vi "Lift_State_Machine.vi"() -> ()   [LabVIEW 2016]
doc: "The state machine for the Lift System.\nDrives the lift forward, then upward, then back, then down to its origin."
uses:
  <vilib>/myRIO/Instrument Drivers/Onboard IO/DIO/typedefs/DIO Reference.ctl
  <vilib>/myRIO/Common/Instrument Driver Framework/Utilities/typedefs/myRIO Generic Hardware Reference.ctl
  <vilib>/myRIO/Common/Instrument Driver Framework/Utilities/typedefs/Hardware Version Enum.ctl
  <vilib>/myRIO/Common/Instrument Driver Framework/Utilities/typedefs/myRIO v1.0 Reference.ctl
  <vilib>/myRIO/Common/Instrument Driver Framework/Utilities/typedefs/Generic FPGA Reference.ctl
  <vilib>/myRIO/Common/Instrument Driver Framework/myRIO v1.0/DIO/typedefs/DIO Channels List.ctl
  <vilib>/myRIO/Common/Instrument Driver Framework/myRIO v1.0/DIO/typedefs/DIO Channels Enum.ctl
  <vilib>/userdefined/High Color/nirio_resource_hc.ctl
  <vilib>/myRIO/Common/Instrument Driver Framework/Utilities/vis/Is FPGA Ref Available.vi
  <vilib>/myRIO/Common/Instrument Driver Framework/roboRIO v1.0/DIO/vis/roboRIO v1.0 Open DIO.vi
  <vilib>/myRIO/Instrument Drivers/Onboard IO/DIO/vis/Write.vi
  <vilib>/myRIO/Instrument Drivers/Onboard IO/DIO/vis/Read.vi
  <vilib>/myRIO/Common/Instrument Driver Framework/Utilities/vis/Validate Channels.vi
  <vilib>/myRIO/Common/Instrument Driver Framework/roboRIO v1.0/DIO/vis/roboRIO v1.0 Reserve DIO.vi
  <vilib>/myRIO/Common/Instrument Driver Framework/roboRIO v1.0/DIO/vis/roboRIO v1.0 Build MUX Configuration DIO.vi
  <vilib>/myRIO/Common/Instrument Driver Framework/roboRIO v1.0/Resource Manager/vis/roboRIO v1.0 Reserve Channel List.vi
  <vilib>/myRIO/Common/Instrument Driver Framework/roboRIO v1.0/Resource Manager/vis/roboRIO v1.0 Create Configuration List.vi
  <vilib>/myRIO/Common/Instrument Driver Framework/roboRIO v1.0/Resource Manager/vis/roboRIO v1.0 Reserve Channel.vi
  <vilib>/myRIO/Common/Instrument Driver Framework/roboRIO v1.0/Resource Manager/vis/roboRIO v1.0 Unreserve Channel.vi
  <vilib>/myRIO/Common/Instrument Driver Framework/roboRIO v1.0/Resource Manager/vis/roboRIO v1.0 Build Mutex Name.vi
  GlobalVI.vi
  <vilib>/Utility/VariantDataType/GetNumericInfo.vi
  <vilib>/Utility/error.llb/Error Cluster From Error Code.vi
  <vilib>/myRIO/Common/Instrument Driver Framework/roboRIO v1.0/roboRIO v1.0 Open.vi
  <vilib>/myRIO/Common/Instrument Driver Framework/Utilities/vis/IO Manager.vi
  <vilib>/myRIO/Common/Instrument Driver Framework/Utilities/vis/Configuration Manager.vi
  <vilib>/myRIO/Common/Instrument Driver Framework/roboRIO v1.0/Resource Manager/vis/roboRIO v1.0 Configure IO.vi
  <vilib>/myRIO/Common/Instrument Driver Framework/myRIO v1.0/myRIO v1.0 Close.vi
  <vilib>/myRIO/Common/Instrument Driver Framework/roboRIO v1.0/DIO/vis/roboRIO v1.0 Read DIO.vi
  <vilib>/myRIO/Common/Instrument Driver Framework/roboRIO v1.0/DIO/vis/roboRIO v1.0 Write DIO.vi
  <vilib>/myRIO/Express VI/Onboard IO/DI/DI Express VI.xnode
  <vilib>/myRIO/Instrument Drivers/Onboard IO/DIO/vis/myRIO DIO Open.xnode
  <vilib>/myRIO/Express VI/Onboard IO/DO/DO Express VI.xnode
  <vilib>/myRIO/Express VI/Onboard Devices/LED/LED Express VI.xnode
  <vilib>/myRIO/Instrument Drivers/Onboard IO/DIO/DIO.lvlib
panel:
  out "DIO/DIO4 (Pin 4)":bool
  out "TrashCanOn":bool
  out "Trash can detection)":bool
  out "B/DIO7 (Pin 25) 4":bool
  out "B/DIO9 (Pin 29) 4":bool
  out "B/DIO8 (Pin 27) 4":bool
  out "B/DIO7 (Pin 25)":bool
  out "B/DIO8 (Pin 27)":bool
  out "B/DIO9 (Pin 29) 2":bool
  in  "runLiftStatemachine":bool
  out "timeoutError":bool
  out "timeoutCounter":u32
  out "timerCount":u32
  out "liftState":i32
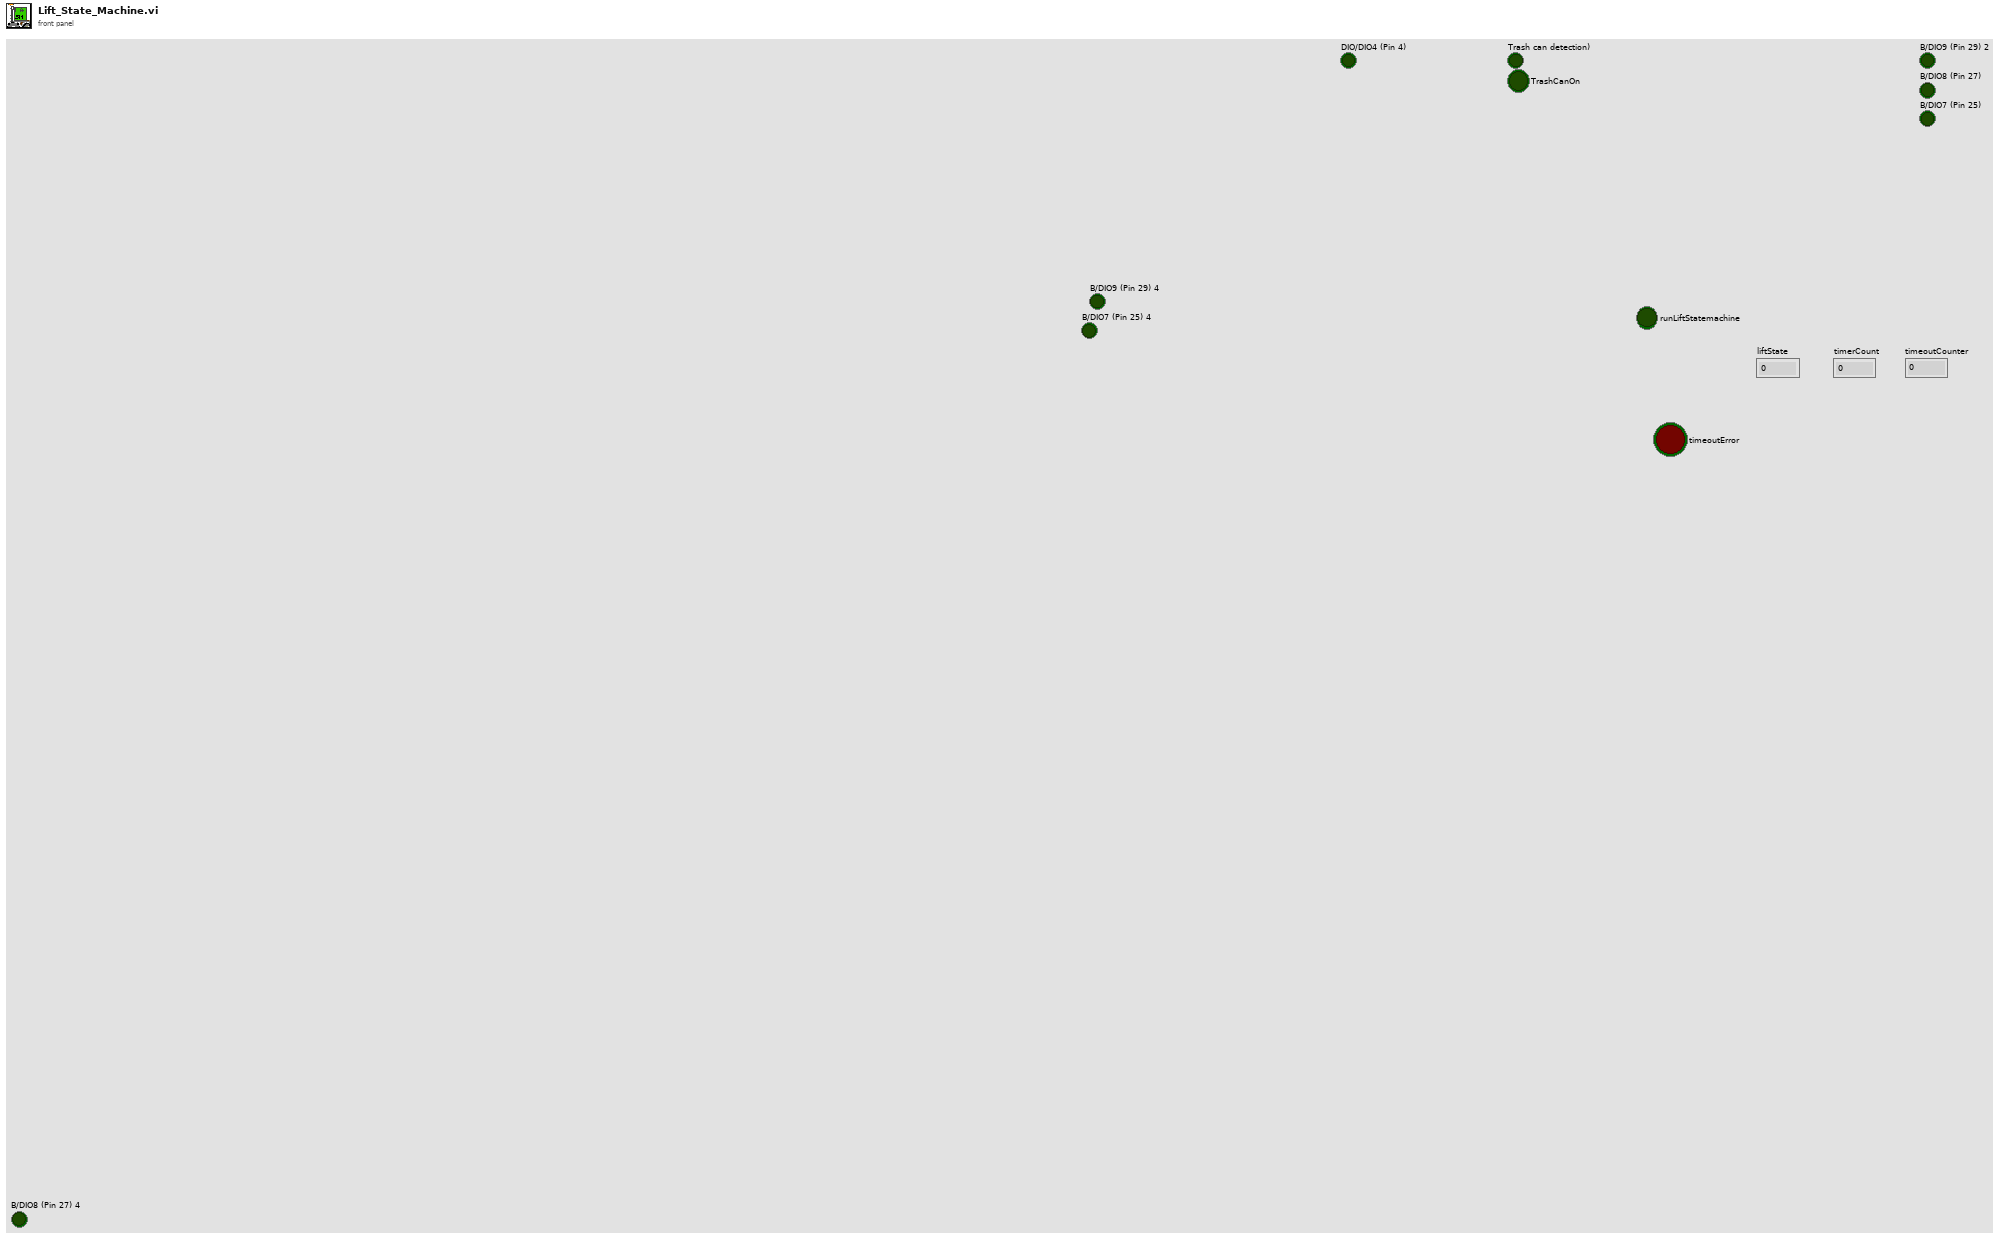
[diagram p1: front panel]
types:
  T1 = typedef "DIO.lvlib/DIO Reference.ctl" = cluster{"myRIO Reference":T2, "DIO Channels List":T6}
  T2 = typedef "myRIO Generic Hardware Reference.ctl" = cluster{"myRIO Model":T3, "myRIO Hardware Reference":T4}
  T3 = typedef "Hardware Version Enum.ctl" = enum16{"Unknown", "myRIO-1900", "myRIO-1950", "roboRIO", "NI ELVIS RIO CM"}
  T4 = typedef "myRIO v1.0 Reference.ctl" = cluster{"Generic FPGA Reference":T5, "Allow multiple opens":bool}
  T5 = typedef "Generic FPGA Reference.ctl" = refnum<k20>
  T6 = typedef "DIO Channels List.ctl" = T7[]
  T7 = typedef "DIO Channels Enum.ctl" = enum16{"Not Connected", "C/DIO0", "C/DIO1", "C/DIO2", "C/DIO3", "C/DIO4", "C/DIO5", "C/DIO6", "C/DIO7", "A/DIO0", "A/DIO1", "A/DIO2", "A/DIO3", "A/DIO4", "A/DIO5", "A/DIO6", "A/DIO7", "A/DIO8", "A/DIO9", "A/DIO10", "A/DIO11", "A/DIO12", "A/DIO13", "A/DIO14", "A/DIO15", "B/DIO0", "B/DIO1", "B/DIO2", "B/DIO3", "B/DIO4", "B/DIO5", "B/DIO6", "B/DIO7", "B/DIO8", "B/DIO9", "B/DIO10", "B/DIO11", "B/DIO12", "B/DIO13", "B/DIO14", "B/DIO15", "LED0", "LED1", "LED2", "LED3", "Button0", "DIO/DIO0", "DIO/DIO1", "DIO/DIO2", "DIO/DIO3", "DIO/DIO4", "DIO/DIO5", "DIO/DIO6", "DIO/DIO7", "DIO/DIO8", "DIO/DIO9", "SPI/CS0", "SPI/CS1", "SPI/CS2", "SPI/CS3", "LED RADIO (Green)", "LED RADIO (Red)", "LED COMM (Green)", "LED COMM (Red)", "LED MODE (Green)", "LED MODE (Red)"}
  T8 = typedef "nirio_resource_hc.ctl" = tag
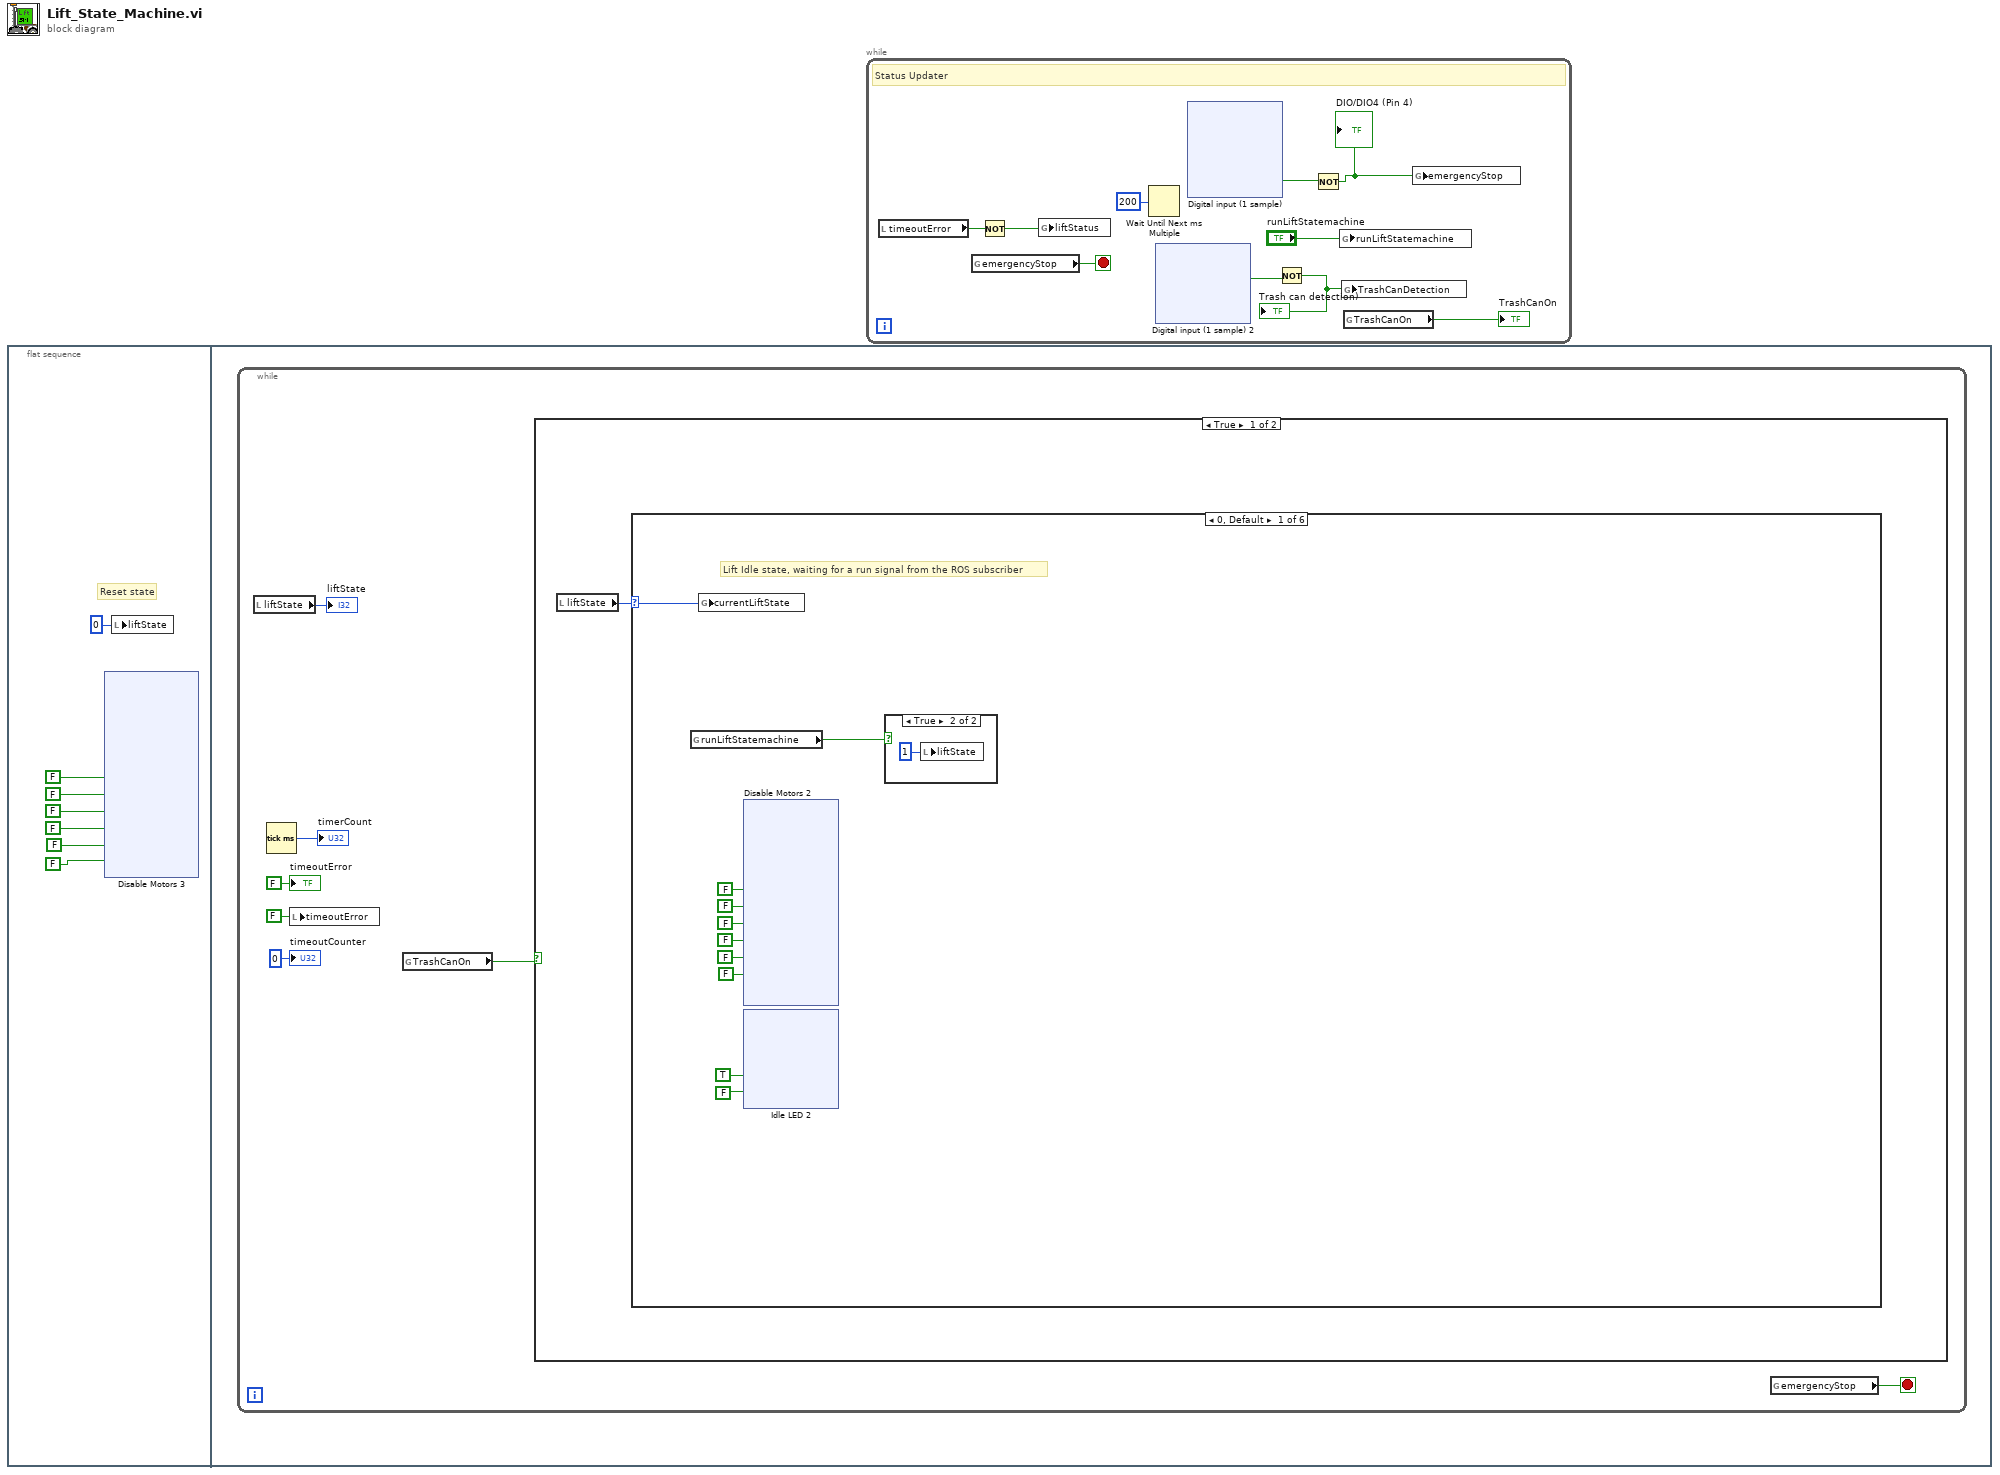
[diagram p0: block diagram]
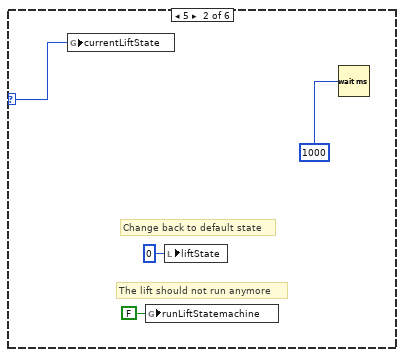
[diagram p3: hidden frame]
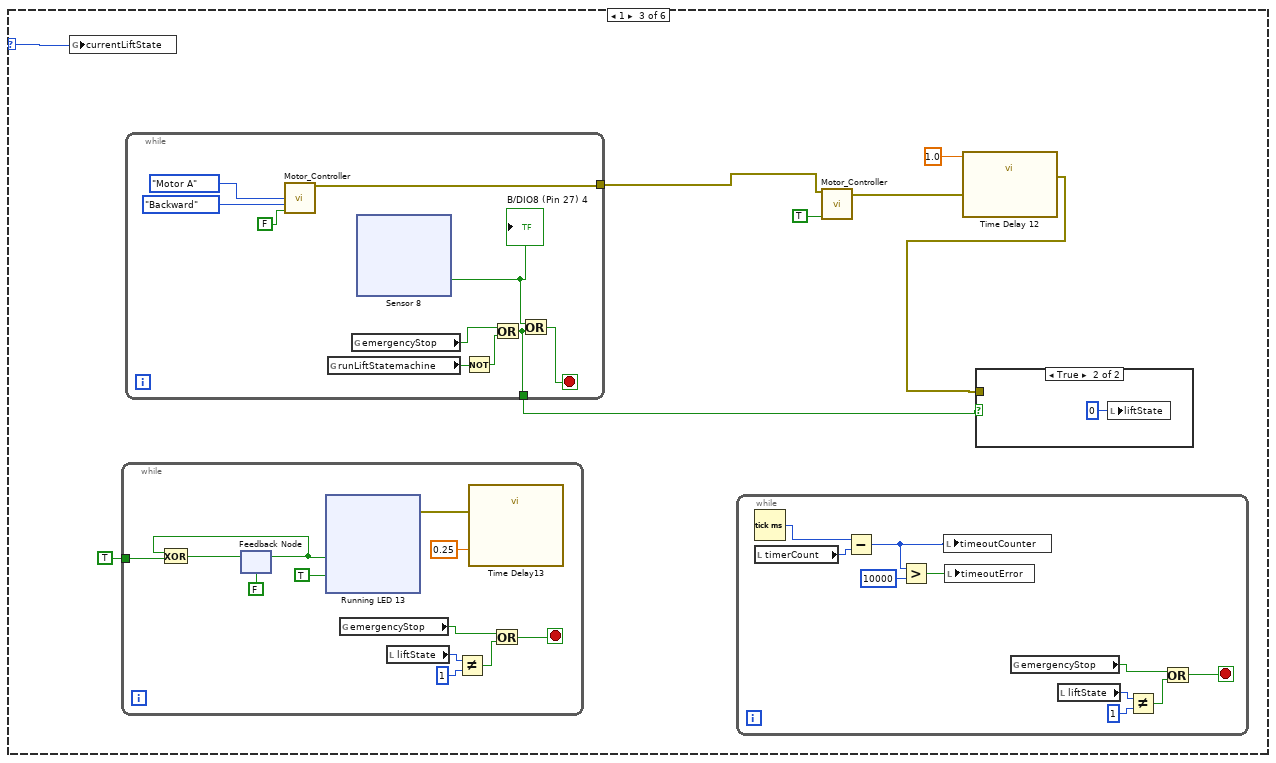
[diagram p4: hidden frame]
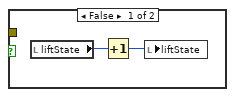
[diagram p5: hidden frame]
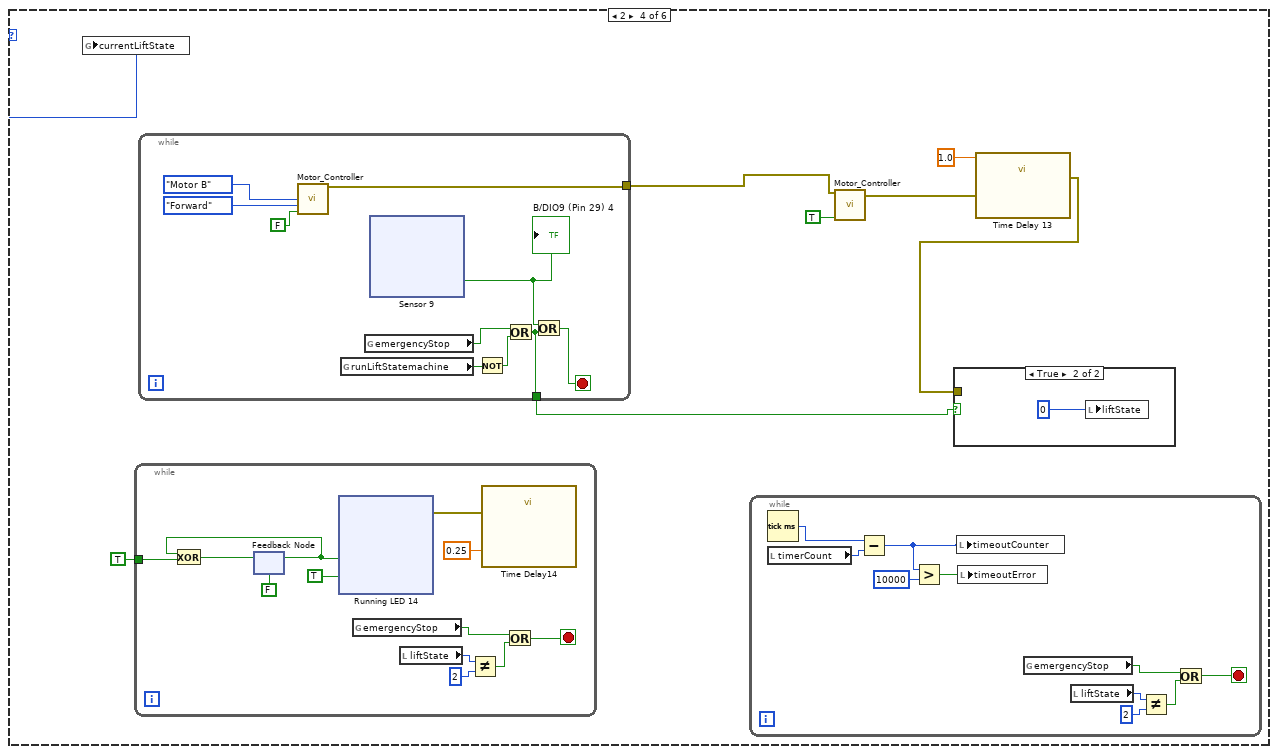
[diagram p6: hidden frame]
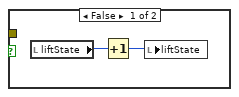
[diagram p7: hidden frame]
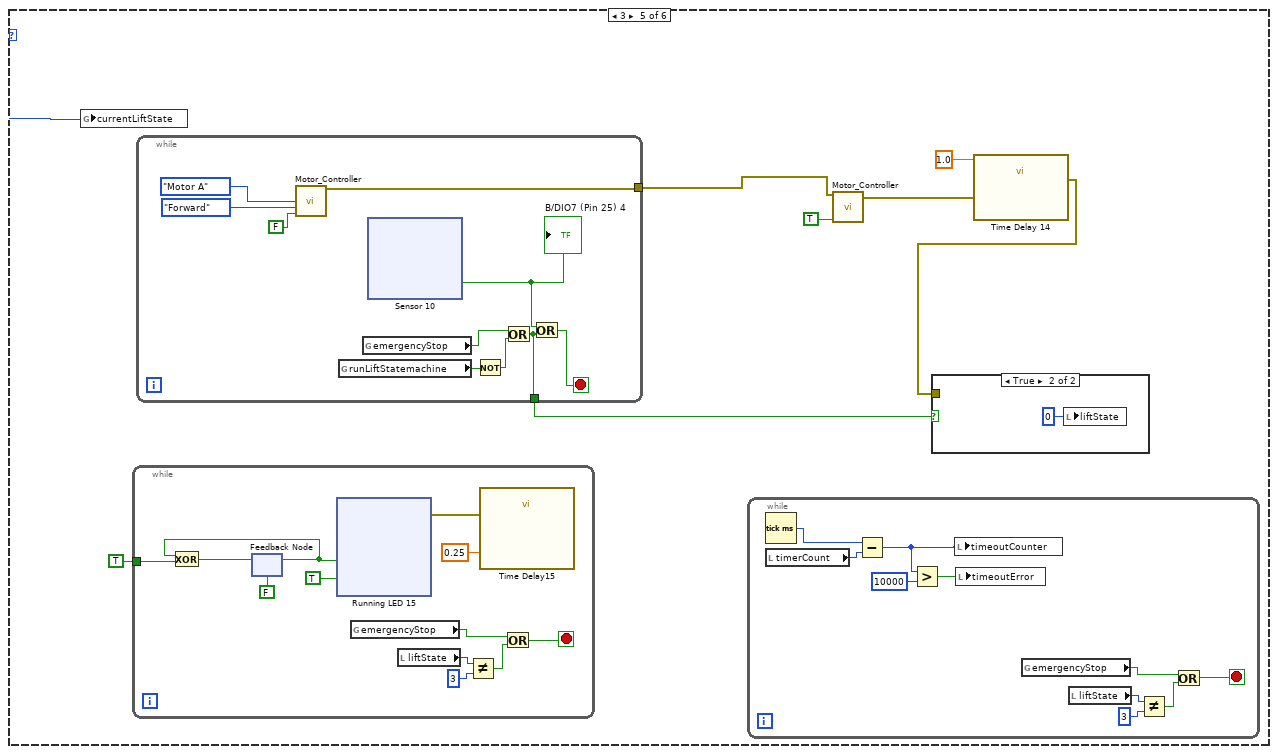
[diagram p8: hidden frame]
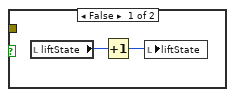
[diagram p9: hidden frame]
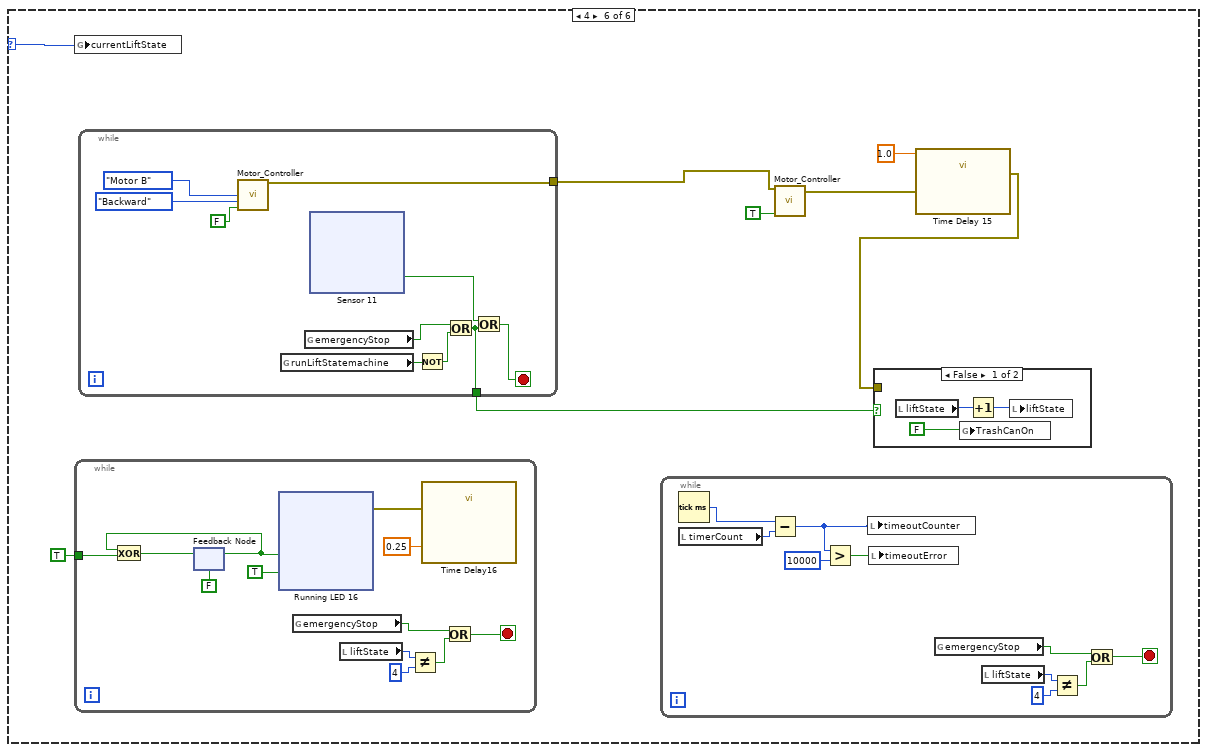
[diagram p10: hidden frame]
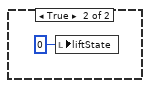
[diagram p11: hidden frame]
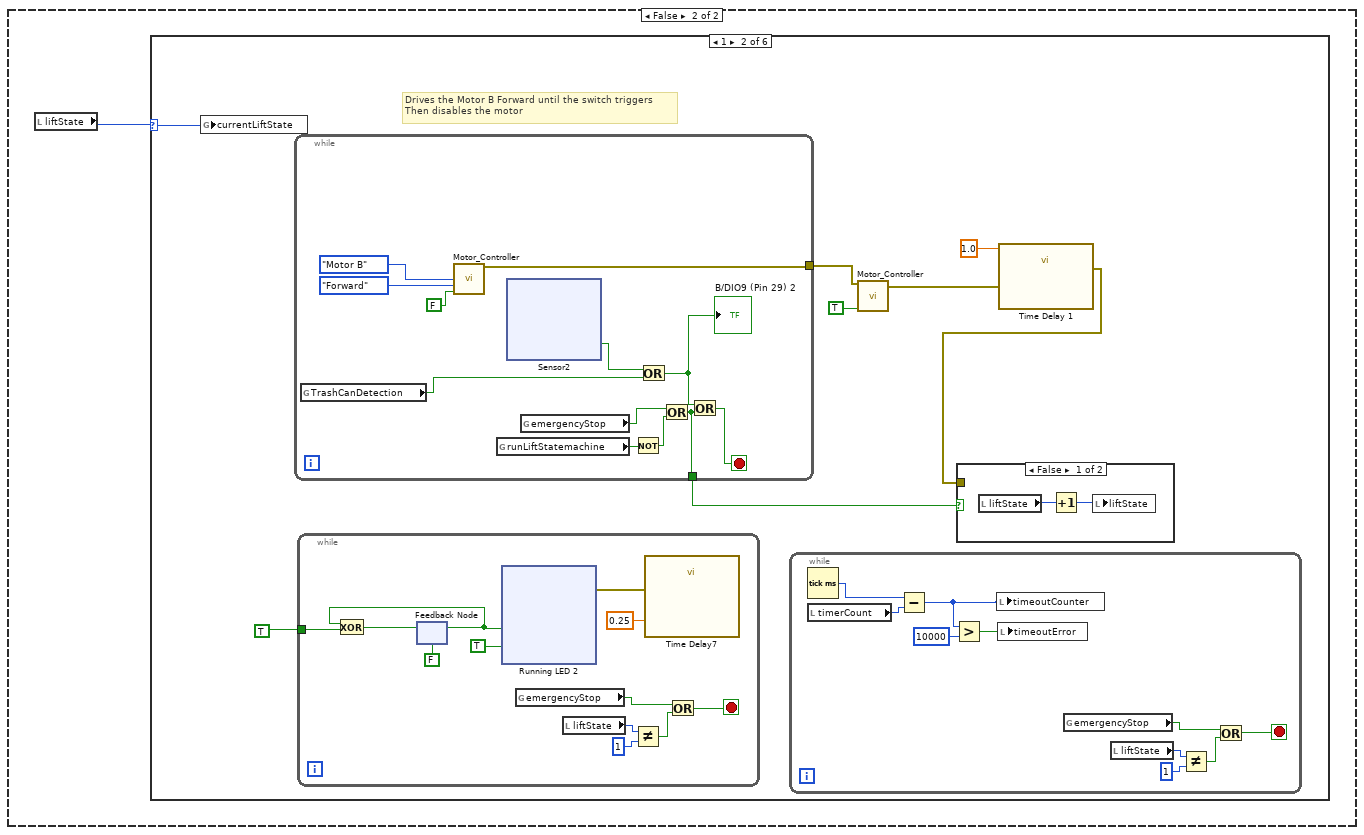
[diagram p12: hidden frame]
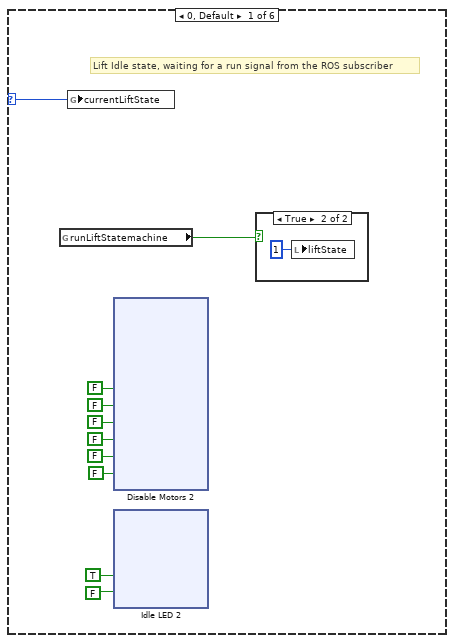
[diagram p13: hidden frame]
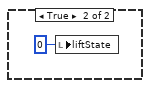
[diagram p15: hidden frame]
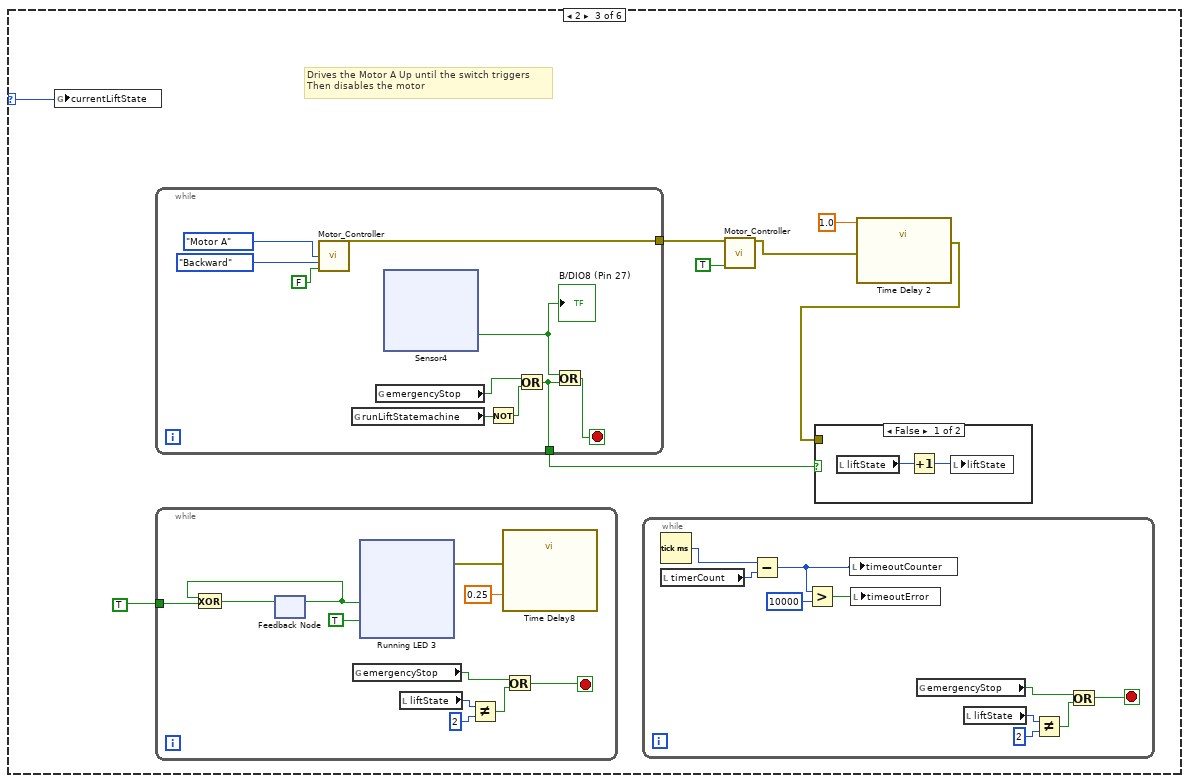
[diagram p16: hidden frame]
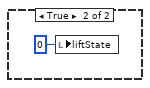
[diagram p17: hidden frame]
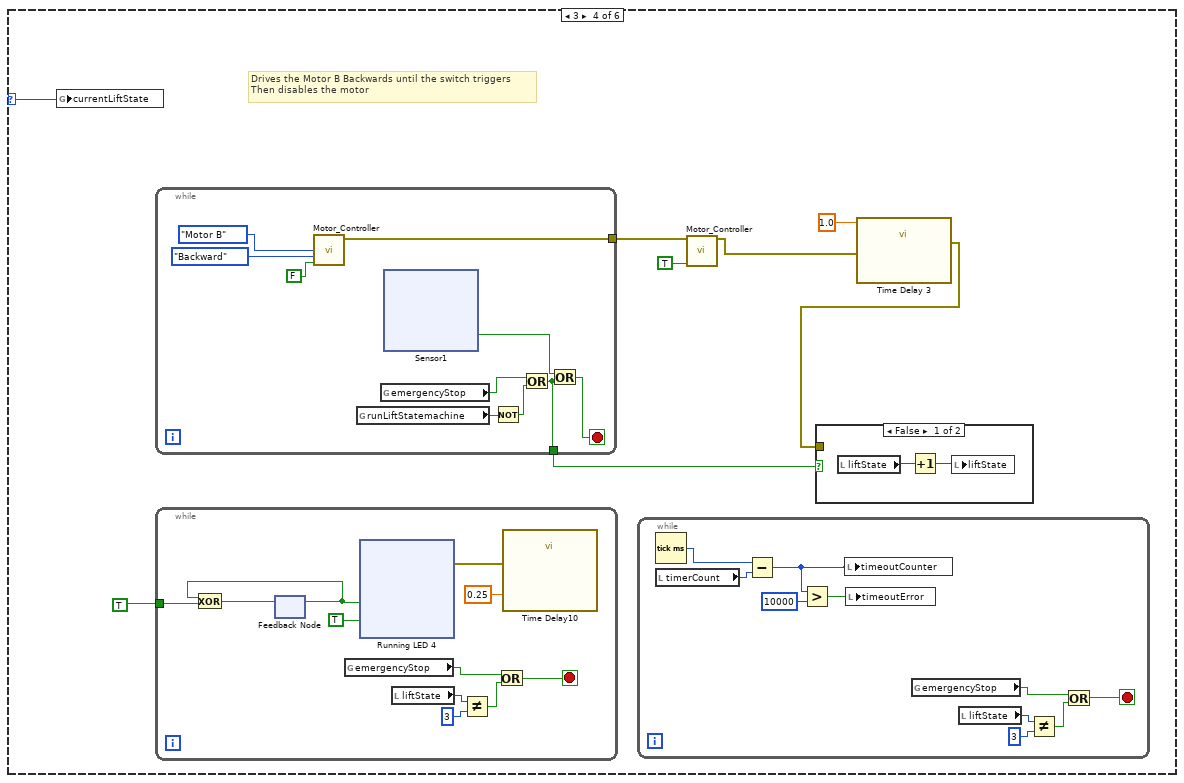
[diagram p18: hidden frame]
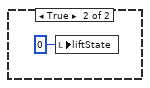
[diagram p19: hidden frame]
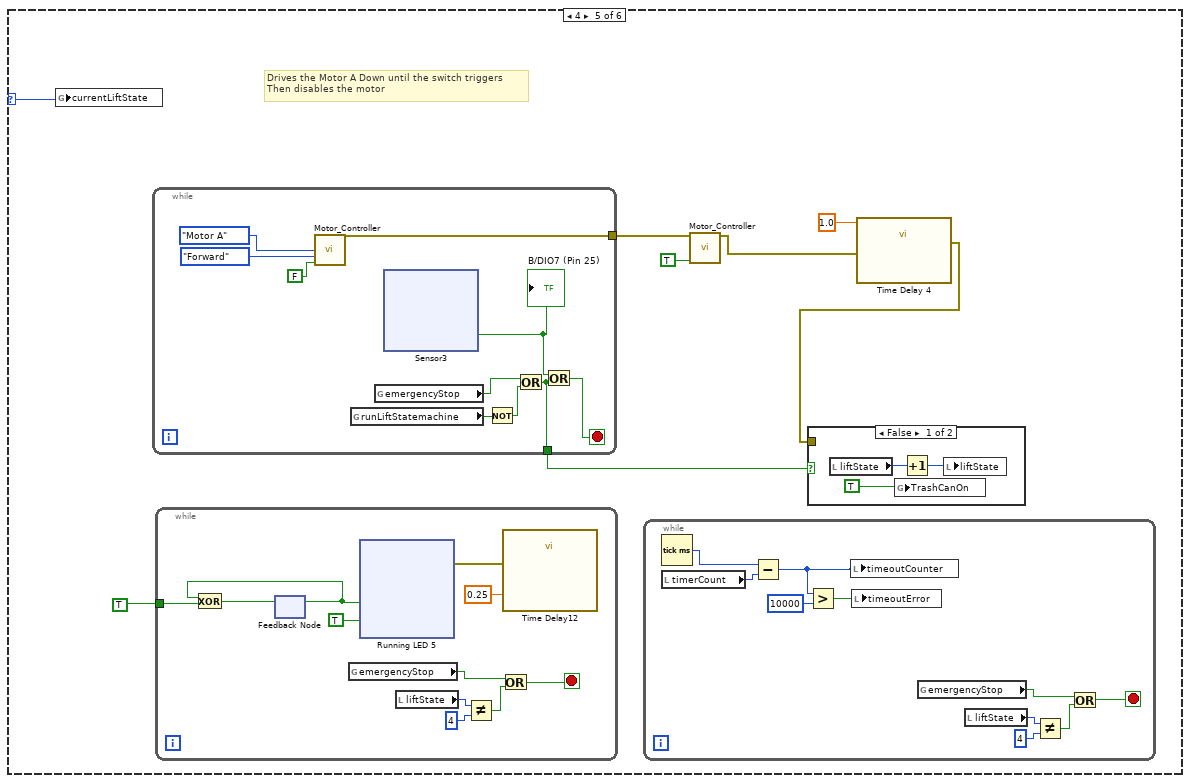
[diagram p20: hidden frame]
diagram:
  n1 = flat-sequence {
    frame #0 {
      # "Reset state"
      n2 = xnode "Disable Motors 3"("IN1 (B/DIO0 (Pin 11))"=FALSE ("IN2 (B/DIO1 (Pin 13))"), "IN2 (B/DIO1 (Pin 13))"=FALSE ("IN3 (B/DIO2 (Pin 15))"), "IN3 (B/DIO2 (Pin 15))"=FALSE ("IN4 (B/DIO3 (Pin 17))"), "IN4 (B/DIO3 (Pin 17))"=FALSE ("ENABLE A (B/DIO13 (Pin 26))"), "ENABLE A (B/DIO13 (Pin 26))"=FALSE ("ENABLE B (B/DIO8 (Pin 27))"), "ENABLE B (B/DIO8 (Pin 27))"=FALSE) -> ()  [unwired: 1 in, 1 out]
      n3 = local write "liftState"(0 ("liftState")) -> ()
    }
    frame #1 {
      n4 = while {
        stop <- w54 stop-if-true
        n5 = local read "liftState"() -> (→"liftState":i32)
        n6 = Tick Count (ms)() -> (millisecond timer value=→"timerCount":u32)
        n7 = local write "timeoutError"(FALSE ("timeoutError")) -> ()
        n8 = global read "GlobalVI.vi" "TrashCanOn"() -> (w48:bool)
        n9 = case shown="True" w48 {
          frame True {
            n10 = local read "liftState"() -> (w55:i32)
            n11 = case shown="0, Default" w55 {
              selector: w55 -> [w56 w145 w154 w263 w375 w489]
              frame 0, Default {
                # "Lift Idle state, waiting for a run signal from the ROS subscriber"
                n12 = global read "GlobalVI.vi" "runLiftStatemachine"() -> (w57:bool)
                n13 = global write "GlobalVI.vi" "currentLiftState"(w56) -> ()
                n14 = xnode "Disable Motors 2"("IN1 (B/DIO0 (Pin 11))"=FALSE, "IN2 (B/DIO1 (Pin 13))"=FALSE, "IN3 (B/DIO2 (Pin 15))"=FALSE, "IN4 (B/DIO3 (Pin 17))"=FALSE, "ENABLE A (B/DIO13 (Pin 26))"=FALSE, "ENABLE B (B/DIO8 (Pin 27))"=FALSE) -> ()  [unwired: 1 in, 1 out]
                n15 = xnode "Idle LED 2"("CommG"=TRUE, "CommR"=FALSE ("CommG")) -> ()  [unwired: 1 in, 1 out]
                n16 = case shown="True" w57 {
                  frame False {
                  }
                  frame True {
                    n17 = local write "liftState"(1 ("liftState")) -> ()
                  }
                }
              }
              frame 5 {
                # "The lift should not run anymore"
                # "Change back to default state"
                n18 = global write "GlobalVI.vi" "currentLiftState"(w145) -> ()
                n19 = global write "GlobalVI.vi" "runLiftStatemachine"(FALSE ("runLiftStatemachine")) -> ()
                n20 = local write "liftState"(0 ("liftState")) -> ()
                n21 = Wait (ms)(milliseconds to wait=u32 1000) -> ()  [unwired: 1 out]
              }
              frame 1 {
                n22 = global write "GlobalVI.vi" "currentLiftState"(w154) -> ()
                n23 = while {
                  tunnel: TRUE ("COMM (Red)") -> [w179]
                  stop <- w169 stop-if-true
                  n24 = feedback #1(FALSE) -> (w177:bool)
                  n25 = Exclusive Or(1:w179, 2:w177) -> (0:w178:bool)
                  n26 = feedback-in #1(w178) -> ()
                  n27 = xnode "Running LED 13"("CommG"=w177, "CommR"=TRUE) -> ("error out"=w174:errorcluster)  [unwired: 1 in]
                  n28 = global read "GlobalVI.vi" "emergencyStop"() -> (w170:bool)
                  n29 = local read "liftState"() -> (w172:i32)
                  n30 = Not Equal?(x=w172, y=1 ("liftState")) -> (x != y?=w171:bool)
                  n31 = call "Time Delay13"("error in (no error)"=w174, "Delay Time (s)"=0.25) -> ()  [unwired: 9 in, 1 out]
                  n32 = Or(x=w170, y=w171) -> (x .or. y?=w169:bool)
                }
                n33 = while {
                  tunnel: [w220] -> w149
                  tunnel: [w221] -> w147
                  stop <- w225 stop-if-true
                  n34 = call "Motor_Controller.vi"("motorSelect"=enum16{"Motor A", "Motor B"}."Motor A", "direction"=enum16{"Forward", "Backward"}."Backward", "stopMotors"=FALSE) -> ("error out"=w220:errorcluster)  [unwired: 12 in]
                  n35 = global read "GlobalVI.vi" "runLiftStatemachine"() -> (w224:bool)
                  n36 = global read "GlobalVI.vi" "emergencyStop"() -> (w222:bool)
                  n37 = xnode "Sensor 8"() -> ("B/DIO8 (Pin 27)"=w216:bool)  [unwired: 1 in, 1 out]
                  "B/DIO8 (Pin 27) 4" <- w216
                  n38 = Not(x=w224) -> (.not. x?=w223:bool)
                  n39 = Or(x=w222, y=w223) -> (x .or. y?=w221:bool)
                  n40 = Or(x=w216, y=w221) -> (x .or. y?=w225:bool)
                }
                n41 = while {
                  stop <- w161 stop-if-true
                  n42 = Tick Count (ms)() -> (millisecond timer value=w167:u32)
                  n43 = local read "timerCount"() -> (w166:u32)
                  n44 = Subtract(x=w167, y=w166) -> (x-y=w158:u32)
                  n45 = Greater?(x=w158, y=u32 10000) -> (0:w159:bool)
                  n46 = local write "timeoutCounter"(w158) -> ()
                  n47 = local write "timeoutError"(w159) -> ()
                  n48 = global read "GlobalVI.vi" "emergencyStop"() -> (w165:bool)
                  n49 = local read "liftState"() -> (w163:i32)
                  n50 = Not Equal?(x=w163, y=1 ("liftState")) -> (x != y?=w164:bool)
                  n51 = Or(x=w165, y=w164) -> (x .or. y?=w161:bool)
                }
                n52 = call "Motor_Controller.vi"("error in (no error)"=w149, "stopMotors"=TRUE) -> ("error out"=w150:errorcluster)  [unwired: 13 in]
                n53 = call "Time Delay 12"("error in (no error)"=w150, "Delay Time (s)"=1.0) -> ("error out"=w148:errorcluster)  [unwired: 9 in]
                n54 = case shown="True" w147 {
                  tunnel: w148 -> [_ _]
                  frame False {
                    n55 = local read "liftState"() -> (w156:i32)
                    n56 = Increment(x=w156) -> (x+1=w155:i32)
                    n57 = local write "liftState"(w155) -> ()
                  }
                  frame True {
                    n58 = local write "liftState"(0 ("liftState")) -> ()
                  }
                }
              }
              frame 2 {
                n59 = global write "GlobalVI.vi" "currentLiftState"(w263) -> ()
                n60 = while {
                  tunnel: TRUE ("COMM (Red)") -> [w293]
                  stop <- w283 stop-if-true
                  n61 = feedback #2(FALSE) -> (w291:bool)
                  n62 = Exclusive Or(1:w293, 2:w291) -> (0:w292:bool)
                  n63 = feedback-in #2(w292) -> ()
                  n64 = xnode "Running LED 14"("CommG"=w291, "CommR"=TRUE) -> ("error out"=w288:errorcluster)  [unwired: 1 in]
                  n65 = global read "GlobalVI.vi" "emergencyStop"() -> (w284:bool)
                  n66 = local read "liftState"() -> (w286:i32)
                  n67 = Not Equal?(x=w286, y=2 ("liftState")) -> (x != y?=w285:bool)
                  n68 = call "Time Delay14"("error in (no error)"=w288, "Delay Time (s)"=0.25) -> ()  [unwired: 9 in, 1 out]
                  n69 = Or(x=w284, y=w285) -> (x .or. y?=w283:bool)
                }
                n70 = while {
                  tunnel: [w334] -> w264
                  tunnel: [w335] -> w261
                  stop <- w339 stop-if-true
                  n71 = call "Motor_Controller.vi"("motorSelect"=enum16{"Motor A", "Motor B"}."Motor B", "direction"=enum16{"Forward", "Backward"}."Forward", "stopMotors"=FALSE) -> ("error out"=w334:errorcluster)  [unwired: 12 in]
                  n72 = global read "GlobalVI.vi" "runLiftStatemachine"() -> (w338:bool)
                  n73 = global read "GlobalVI.vi" "emergencyStop"() -> (w336:bool)
                  n74 = xnode "Sensor 9"() -> ("B/DIO9 (Pin 29)"=w330:bool)  [unwired: 1 in, 1 out]
                  "B/DIO9 (Pin 29) 4" <- w330
                  n75 = Not(x=w338) -> (.not. x?=w337:bool)
                  n76 = Or(x=w336, y=w337) -> (x .or. y?=w335:bool)
                  n77 = Or(x=w330, y=w335) -> (x .or. y?=w339:bool)
                }
                n78 = while {
                  stop <- w275 stop-if-true
                  n79 = Tick Count (ms)() -> (millisecond timer value=w281:u32)
                  n80 = local read "timerCount"() -> (w280:u32)
                  n81 = Subtract(x=w281, y=w280) -> (x-y=w272:u32)
                  n82 = Greater?(x=w272, y=u32 10000) -> (0:w273:bool)
                  n83 = local write "timeoutCounter"(w272) -> ()
                  n84 = local write "timeoutError"(w273) -> ()
                  n85 = global read "GlobalVI.vi" "emergencyStop"() -> (w279:bool)
                  n86 = local read "liftState"() -> (w277:i32)
                  n87 = Not Equal?(x=w277, y=2 ("liftState")) -> (x != y?=w278:bool)
                  n88 = Or(x=w279, y=w278) -> (x .or. y?=w275:bool)
                }
                n89 = call "Motor_Controller.vi"("error in (no error)"=w264, "stopMotors"=TRUE) -> ("error out"=w265:errorcluster)  [unwired: 13 in]
                n90 = call "Time Delay 13"("error in (no error)"=w265, "Delay Time (s)"=1.0) -> ("error out"=w262:errorcluster)  [unwired: 9 in]
                n91 = case shown="True" w261 {
                  tunnel: w262 -> [_ _]
                  frame False {
                    n92 = local read "liftState"() -> (w270:i32)
                    n93 = Increment(x=w270) -> (x+1=w269:i32)
                    n94 = local write "liftState"(w269) -> ()
                  }
                  frame True {
                    n95 = local write "liftState"(0 ("liftState")) -> ()
                  }
                }
              }
              frame 3 {
                n96 = global write "GlobalVI.vi" "currentLiftState"(w375) -> ()
                n97 = while {
                  tunnel: TRUE ("COMM (Red)") -> [w407]
                  stop <- w397 stop-if-true
                  n98 = feedback #3(FALSE) -> (w405:bool)
                  n99 = Exclusive Or(1:w407, 2:w405) -> (0:w406:bool)
                  n100 = feedback-in #3(w406) -> ()
                  n101 = xnode "Running LED 15"("CommG"=w405, "CommR"=TRUE) -> ("error out"=w402:errorcluster)  [unwired: 1 in]
                  n102 = global read "GlobalVI.vi" "emergencyStop"() -> (w398:bool)
                  n103 = local read "liftState"() -> (w400:i32)
                  n104 = Not Equal?(x=w400, y=3 ("liftState")) -> (x != y?=w399:bool)
                  n105 = call "Time Delay15"("error in (no error)"=w402, "Delay Time (s)"=0.25) -> ()  [unwired: 9 in, 1 out]
                  n106 = Or(x=w398, y=w399) -> (x .or. y?=w397:bool)
                }
                n107 = while {
                  tunnel: [w448] -> w377
                  tunnel: [w449] -> w376
                  stop <- w453 stop-if-true
                  n108 = call "Motor_Controller.vi"("motorSelect"=enum16{"Motor A", "Motor B"}."Motor A", "direction"=enum16{"Forward", "Backward"}."Forward", "stopMotors"=FALSE) -> ("error out"=w448:errorcluster)  [unwired: 12 in]
                  n109 = global read "GlobalVI.vi" "runLiftStatemachine"() -> (w452:bool)
                  n110 = global read "GlobalVI.vi" "emergencyStop"() -> (w450:bool)
                  n111 = xnode "Sensor 10"() -> ("B/DIO7 (Pin 25)"=w444:bool)  [unwired: 1 in, 1 out]
                  "B/DIO7 (Pin 25) 4" <- w444
                  n112 = Not(x=w452) -> (.not. x?=w451:bool)
                  n113 = Or(x=w450, y=w451) -> (x .or. y?=w449:bool)
                  n114 = Or(x=w444, y=w449) -> (x .or. y?=w453:bool)
                }
                n115 = while {
                  stop <- w389 stop-if-true
                  n116 = Tick Count (ms)() -> (millisecond timer value=w395:u32)
                  n117 = local read "timerCount"() -> (w394:u32)
                  n118 = Subtract(x=w395, y=w394) -> (x-y=w386:u32)
                  n119 = Greater?(x=w386, y=u32 10000) -> (0:w387:bool)
                  n120 = local write "timeoutCounter"(w386) -> ()
                  n121 = local write "timeoutError"(w387) -> ()
                  n122 = global read "GlobalVI.vi" "emergencyStop"() -> (w393:bool)
                  n123 = local read "liftState"() -> (w391:i32)
                  n124 = Not Equal?(x=w391, y=3 ("liftState")) -> (x != y?=w392:bool)
                  n125 = Or(x=w393, y=w392) -> (x .or. y?=w389:bool)
                }
                n126 = call "Motor_Controller.vi"("error in (no error)"=w377, "stopMotors"=TRUE) -> ("error out"=w378:errorcluster)  [unwired: 13 in]
                n127 = call "Time Delay 14"("error in (no error)"=w378, "Delay Time (s)"=1.0) -> ("error out"=w380:errorcluster)  [unwired: 9 in]
                n128 = case shown="True" w376 {
                  tunnel: w380 -> [_ _]
                  frame False {
                    n129 = local read "liftState"() -> (w384:i32)
                    n130 = Increment(x=w384) -> (x+1=w383:i32)
                    n131 = local write "liftState"(w383) -> ()
                  }
                  frame True {
                    n132 = local write "liftState"(0 ("liftState")) -> ()
                  }
                }
              }
              frame 4 {
                n133 = global write "GlobalVI.vi" "currentLiftState"(w489) -> ()
                n134 = while {
                  tunnel: TRUE ("COMM (Red)") -> [w522]
                  stop <- w512 stop-if-true
                  n135 = feedback #4(FALSE) -> (w520:bool)
                  n136 = Exclusive Or(1:w522, 2:w520) -> (0:w521:bool)
                  n137 = feedback-in #4(w521) -> ()
                  n138 = xnode "Running LED 16"("CommG"=w520, "CommR"=TRUE) -> ("error out"=w517:errorcluster)  [unwired: 1 in]
                  n139 = global read "GlobalVI.vi" "emergencyStop"() -> (w513:bool)
                  n140 = local read "liftState"() -> (w515:i32)
                  n141 = Not Equal?(x=w515, y=4 ("liftState")) -> (x != y?=w514:bool)
                  n142 = call "Time Delay16"("error in (no error)"=w517, "Delay Time (s)"=0.25) -> ()  [unwired: 9 in, 1 out]
                  n143 = Or(x=w513, y=w514) -> (x .or. y?=w512:bool)
                }
                n144 = while {
                  tunnel: [w563] -> w491
                  tunnel: [w564] -> w490
                  stop <- w568 stop-if-true
                  n145 = call "Motor_Controller.vi"("motorSelect"=enum16{"Motor A", "Motor B"}."Motor B", "direction"=enum16{"Forward", "Backward"}."Backward", "stopMotors"=FALSE) -> ("error out"=w563:errorcluster)  [unwired: 12 in]
                  n146 = global read "GlobalVI.vi" "runLiftStatemachine"() -> (w567:bool)
                  n147 = global read "GlobalVI.vi" "emergencyStop"() -> (w565:bool)
                  n148 = xnode "Sensor 11"() -> ("B/DIO10 (Pin 31)"=w559:bool)  [unwired: 1 in, 1 out]
                  n149 = Not(x=w567) -> (.not. x?=w566:bool)
                  n150 = Or(x=w565, y=w566) -> (x .or. y?=w564:bool)
                  n151 = Or(x=w559, y=w564) -> (x .or. y?=w568:bool)
                }
                n152 = while {
                  stop <- w504 stop-if-true
                  n153 = Tick Count (ms)() -> (millisecond timer value=w510:u32)
                  n154 = local read "timerCount"() -> (w509:u32)
                  n155 = Subtract(x=w510, y=w509) -> (x-y=w501:u32)
                  n156 = Greater?(x=w501, y=u32 10000) -> (0:w502:bool)
                  n157 = local write "timeoutCounter"(w501) -> ()
                  n158 = local write "timeoutError"(w502) -> ()
                  n159 = global read "GlobalVI.vi" "emergencyStop"() -> (w508:bool)
                  n160 = local read "liftState"() -> (w506:i32)
                  n161 = Not Equal?(x=w506, y=4 ("liftState")) -> (x != y?=w507:bool)
                  n162 = Or(x=w508, y=w507) -> (x .or. y?=w504:bool)
                }
                n163 = call "Motor_Controller.vi"("error in (no error)"=w491, "stopMotors"=TRUE) -> ("error out"=w492:errorcluster)  [unwired: 13 in]
                n164 = call "Time Delay 15"("error in (no error)"=w492, "Delay Time (s)"=1.0) -> ("error out"=w494:errorcluster)  [unwired: 9 in]
                n165 = case shown="False" w490 {
                  tunnel: w494 -> [_ _]
                  frame False {
                    n166 = local read "liftState"() -> (w499:i32)
                    n167 = global write "GlobalVI.vi" "TrashCanOn"(FALSE ("TrashCanOn")) -> ()
                    n168 = Increment(x=w499) -> (x+1=w498:i32)
                    n169 = local write "liftState"(w498) -> ()
                  }
                  frame True {
                    n170 = local write "liftState"(0 ("liftState")) -> ()
                  }
                }
              }
            }
          }
          frame False {
            n171 = local read "liftState"() -> (w604:i32)
            n172 = case shown="1" w604 {
              selector: w604 -> [w605 w692 w808 w921 w1034 w1150]
              frame 0, Default {
                # "Lift Idle state, waiting for a run signal from the ROS subscriber"
                n173 = global read "GlobalVI.vi" "runLiftStatemachine"() -> (w606:bool)
                n174 = global write "GlobalVI.vi" "currentLiftState"(w605) -> ()
                n175 = xnode "Disable Motors 2"("IN1 (B/DIO0 (Pin 11))"=FALSE, "IN2 (B/DIO1 (Pin 13))"=FALSE, "IN3 (B/DIO2 (Pin 15))"=FALSE, "IN4 (B/DIO3 (Pin 17))"=FALSE, "ENABLE A (B/DIO13 (Pin 26))"=FALSE, "ENABLE B (B/DIO8 (Pin 27))"=FALSE) -> ()  [unwired: 1 in, 1 out]
                n176 = xnode "Idle LED 2"("CommG"=TRUE, "CommR"=FALSE ("CommG")) -> ()  [unwired: 1 in, 1 out]
                n177 = case shown="True" w606 {
                  frame False {
                  }
                  frame True {
                    n178 = local write "liftState"(1 ("liftState")) -> ()
                  }
                }
              }
              frame 1 {
                # "Drives the Motor B Forward until the switch triggers\nThen disables the motor"
                n179 = global write "GlobalVI.vi" "currentLiftState"(w692) -> ()
                n180 = while {
                  tunnel: [w767] -> w693
                  tunnel: [w768] -> w696
                  stop <- w772 stop-if-true
                  n181 = global read "GlobalVI.vi" "TrashCanDetection"() -> (w761:bool)
                  n182 = call "Motor_Controller.vi"("motorSelect"=enum16{"Motor A", "Motor B"}."Motor B", "direction"=enum16{"Forward", "Backward"}."Forward", "stopMotors"=FALSE) -> ("error out"=w767:errorcluster)  [unwired: 12 in]
                  n183 = global read "GlobalVI.vi" "runLiftStatemachine"() -> (w771:bool)
                  n184 = xnode "Sensor2"() -> ("B/DIO9 (Pin 29)"=w762:bool)  [unwired: 1 in, 1 out]
                  n185 = global read "GlobalVI.vi" "emergencyStop"() -> (w769:bool)
                  n186 = Not(x=w771) -> (.not. x?=w770:bool)
                  n187 = Or(x=w762, y=w761) -> (x .or. y?=w763:bool)
                  "B/DIO9 (Pin 29) 2" <- w763
                  n188 = Or(x=w769, y=w770) -> (x .or. y?=w768:bool)
                  n189 = Or(x=w763, y=w768) -> (x .or. y?=w772:bool)
                }
                n190 = while {
                  tunnel: TRUE ("COMM (Red)") -> [w724]
                  stop <- w714 stop-if-true
                  n191 = feedback #5(FALSE) -> (w722:bool)
                  n192 = Exclusive Or(1:w724, 2:w722) -> (0:w723:bool)
                  n193 = feedback-in #5(w723) -> ()
                  n194 = xnode "Running LED 2"("CommG"=w722, "CommR"=TRUE) -> ("error out"=w719:errorcluster)  [unwired: 1 in]
                  n195 = global read "GlobalVI.vi" "emergencyStop"() -> (w715:bool)
                  n196 = local read "liftState"() -> (w717:i32)
                  n197 = Not Equal?(x=w717, y=1 ("liftState")) -> (x != y?=w716:bool)
                  n198 = call "Time Delay7"("error in (no error)"=w719, "Delay Time (s)"=0.25) -> ()  [unwired: 9 in, 1 out]
                  n199 = Or(x=w715, y=w716) -> (x .or. y?=w714:bool)
                }
                n200 = while {
                  stop <- w703 stop-if-true
                  n201 = Tick Count (ms)() -> (millisecond timer value=w709:u32)
                  n202 = local read "timerCount"() -> (w708:u32)
                  n203 = Subtract(x=w709, y=w708) -> (x-y=w700:u32)
                  n204 = Greater?(x=w700, y=u32 10000) -> (0:w701:bool)
                  n205 = local write "timeoutCounter"(w700) -> ()
                  n206 = local write "timeoutError"(w701) -> ()
                  n207 = global read "GlobalVI.vi" "emergencyStop"() -> (w707:bool)
                  n208 = local read "liftState"() -> (w705:i32)
                  n209 = Not Equal?(x=w705, y=1 ("liftState")) -> (x != y?=w706:bool)
                  n210 = Or(x=w707, y=w706) -> (x .or. y?=w703:bool)
                }
                n211 = call "Motor_Controller.vi"("error in (no error)"=w693, "stopMotors"=TRUE) -> ("error out"=w694:errorcluster)  [unwired: 13 in]
                n212 = call "Time Delay 1"("error in (no error)"=w694, "Delay Time (s)"=1.0) -> ("error out"=w697:errorcluster)  [unwired: 9 in]
                n213 = case shown="False" w696 {
                  tunnel: w697 -> [_ _]
                  frame False {
                    n214 = local read "liftState"() -> (w711:i32)
                    n215 = Increment(x=w711) -> (x+1=w710:i32)
                    n216 = local write "liftState"(w710) -> ()
                  }
                  frame True {
                    n217 = local write "liftState"(0 ("liftState")) -> ()
                  }
                }
              }
              frame 2 {
                # "Drives the Motor A Up until the switch triggers\nThen disables the motor"
                n218 = global write "GlobalVI.vi" "currentLiftState"(w808) -> ()
                n219 = while {
                  tunnel: [w881] -> w812
                  tunnel: [w878] -> w810
                  stop <- w882 stop-if-true
                  n220 = call "Motor_Controller.vi"("motorSelect"=enum16{"Motor A", "Motor B"}."Motor A", "direction"=enum16{"Forward", "Backward"}."Backward", "stopMotors"=FALSE) -> ("error out"=w878:errorcluster)  [unwired: 12 in]
                  n221 = global read "GlobalVI.vi" "runLiftStatemachine"() -> (w885:bool)
                  n222 = global read "GlobalVI.vi" "emergencyStop"() -> (w883:bool)
                  n223 = xnode "Sensor4"() -> ("B/DIO8 (Pin 27)"=w876:bool)  [unwired: 1 in, 1 out]
                  "B/DIO8 (Pin 27)" <- w876
                  n224 = Not(x=w885) -> (.not. x?=w884:bool)
                  n225 = Or(x=w883, y=w884) -> (x .or. y?=w881:bool)
                  n226 = Or(x=w876, y=w881) -> (x .or. y?=w882:bool)
                }
                n227 = while {
                  tunnel: TRUE ("COMM (Red)") -> [w839]
                  stop <- w829 stop-if-true
                  n228 = feedback #6() -> (w837:bool)  [unwired: 1 in]
                  n229 = Exclusive Or(1:w839, 2:w837) -> (0:w838:bool)
                  n230 = feedback-in #6(w838) -> ()
                  n231 = global read "GlobalVI.vi" "emergencyStop"() -> (w830:bool)
                  n232 = xnode "Running LED 3"("CommG"=w837, "CommR"=TRUE) -> ("error out"=w834:errorcluster)  [unwired: 1 in]
                  n233 = local read "liftState"() -> (w832:i32)
                  n234 = Not Equal?(x=w832, y=2 ("liftState")) -> (x != y?=w831:bool)
                  n235 = call "Time Delay8"("error in (no error)"=w834, "Delay Time (s)"=0.25) -> ()  [unwired: 9 in, 1 out]
                  n236 = Or(x=w830, y=w831) -> (x .or. y?=w829:bool)
                }
                n237 = while {
                  stop <- w819 stop-if-true
                  n238 = Tick Count (ms)() -> (millisecond timer value=w825:u32)
                  n239 = local read "timerCount"() -> (w824:u32)
                  n240 = Subtract(x=w825, y=w824) -> (x-y=w816:u32)
                  n241 = Greater?(x=w816, y=u32 10000) -> (0:w817:bool)
                  n242 = local write "timeoutCounter"(w816) -> ()
                  n243 = local write "timeoutError"(w817) -> ()
                  n244 = global read "GlobalVI.vi" "emergencyStop"() -> (w823:bool)
                  n245 = local read "liftState"() -> (w821:i32)
                  n246 = Not Equal?(x=w821, y=2 ("liftState")) -> (x != y?=w822:bool)
                  n247 = Or(x=w823, y=w822) -> (x .or. y?=w819:bool)
                }
                n248 = call "Motor_Controller.vi"("error in (no error)"=w810, "stopMotors"=TRUE) -> ("error out"=w809:errorcluster)  [unwired: 13 in]
                n249 = call "Time Delay 2"("error in (no error)"=w809, "Delay Time (s)"=1.0) -> ("error out"=w813:errorcluster)  [unwired: 9 in]
                n250 = case shown="False" w812 {
                  tunnel: w813 -> [_ _]
                  frame False {
                    n251 = local read "liftState"() -> (w827:i32)
                    n252 = Increment(x=w827) -> (x+1=w826:i32)
                    n253 = local write "liftState"(w826) -> ()
                  }
                  frame True {
                    n254 = local write "liftState"(0 ("liftState")) -> ()
                  }
                }
              }
              frame 3 {
                # "Drives the Motor B Backwards until the switch triggers\nThen disables the motor"
                n255 = global write "GlobalVI.vi" "currentLiftState"(w921) -> ()
                n256 = while {
                  tunnel: [w994] -> w925
                  tunnel: [w991] -> w923
                  stop <- w995 stop-if-true
                  n257 = call "Motor_Controller.vi"("motorSelect"=enum16{"Motor A", "Motor B"}."Motor B", "direction"=enum16{"Forward", "Backward"}."Backward", "stopMotors"=FALSE) -> ("error out"=w991:errorcluster)  [unwired: 12 in]
                  n258 = global read "GlobalVI.vi" "runLiftStatemachine"() -> (w998:bool)
                  n259 = global read "GlobalVI.vi" "emergencyStop"() -> (w996:bool)
                  n260 = xnode "Sensor1"() -> ("B/DIO10 (Pin 31)"=w989:bool)  [unwired: 1 in, 1 out]
                  n261 = Not(x=w998) -> (.not. x?=w997:bool)
                  n262 = Or(x=w996, y=w997) -> (x .or. y?=w994:bool)
                  n263 = Or(x=w989, y=w994) -> (x .or. y?=w995:bool)
                }
                n264 = while {
                  tunnel: TRUE ("COMM (Red)") -> [w952]
                  stop <- w942 stop-if-true
                  n265 = feedback #7() -> (w950:bool)  [unwired: 1 in]
                  n266 = Exclusive Or(1:w952, 2:w950) -> (0:w951:bool)
                  n267 = feedback-in #7(w951) -> ()
                  n268 = global read "GlobalVI.vi" "emergencyStop"() -> (w943:bool)
                  n269 = xnode "Running LED 4"("CommG"=w950, "CommR"=TRUE) -> ("error out"=w947:errorcluster)  [unwired: 1 in]
                  n270 = local read "liftState"() -> (w945:i32)
                  n271 = Not Equal?(x=w945, y=3 ("liftState")) -> (x != y?=w944:bool)
                  n272 = Or(x=w943, y=w944) -> (x .or. y?=w942:bool)
                  n273 = call "Time Delay10"("error in (no error)"=w947, "Delay Time (s)"=0.25) -> ()  [unwired: 9 in, 1 out]
                }
                n274 = while {
                  stop <- w932 stop-if-true
                  n275 = Tick Count (ms)() -> (millisecond timer value=w938:u32)
                  n276 = local read "timerCount"() -> (w937:u32)
                  n277 = Subtract(x=w938, y=w937) -> (x-y=w929:u32)
                  n278 = Greater?(x=w929, y=u32 10000) -> (0:w930:bool)
                  n279 = local write "timeoutCounter"(w929) -> ()
                  n280 = local write "timeoutError"(w930) -> ()
                  n281 = global read "GlobalVI.vi" "emergencyStop"() -> (w936:bool)
                  n282 = local read "liftState"() -> (w934:i32)
                  n283 = Not Equal?(x=w934, y=3 ("liftState")) -> (x != y?=w935:bool)
                  n284 = Or(x=w936, y=w935) -> (x .or. y?=w932:bool)
                }
                n285 = call "Motor_Controller.vi"("error in (no error)"=w923, "stopMotors"=TRUE) -> ("error out"=w922:errorcluster)  [unwired: 13 in]
                n286 = call "Time Delay 3"("error in (no error)"=w922, "Delay Time (s)"=1.0) -> ("error out"=w926:errorcluster)  [unwired: 9 in]
                n287 = case shown="False" w925 {
                  tunnel: w926 -> [_ _]
                  frame False {
                    n288 = local read "liftState"() -> (w940:i32)
                    n289 = Increment(x=w940) -> (x+1=w939:i32)
                    n290 = local write "liftState"(w939) -> ()
                  }
                  frame True {
                    n291 = local write "liftState"(0 ("liftState")) -> ()
                  }
                }
              }
              frame 4 {
                # "Drives the Motor A Down until the switch triggers\nThen disables the motor"
                n292 = global write "GlobalVI.vi" "currentLiftState"(w1034) -> ()
                n293 = while {
                  tunnel: [w1108] -> w1039
                  tunnel: [w1105] -> w1036
                  stop <- w1109 stop-if-true
                  n294 = call "Motor_Controller.vi"("motorSelect"=enum16{"Motor A", "Motor B"}."Motor A", "direction"=enum16{"Forward", "Backward"}."Forward", "stopMotors"=FALSE) -> ("error out"=w1105:errorcluster)  [unwired: 12 in]
                  n295 = global read "GlobalVI.vi" "runLiftStatemachine"() -> (w1112:bool)
                  n296 = global read "GlobalVI.vi" "emergencyStop"() -> (w1110:bool)
                  n297 = xnode "Sensor3"() -> ("B/DIO7 (Pin 25)"=w1103:bool)  [unwired: 1 in, 1 out]
                  "B/DIO7 (Pin 25)" <- w1103
                  n298 = Not(x=w1112) -> (.not. x?=w1111:bool)
                  n299 = Or(x=w1110, y=w1111) -> (x .or. y?=w1108:bool)
                  n300 = Or(x=w1103, y=w1108) -> (x .or. y?=w1109:bool)
                }
                n301 = while {
                  tunnel: TRUE ("COMM (Red)") -> [w1066]
                  stop <- w1056 stop-if-true
                  n302 = feedback #8() -> (w1064:bool)  [unwired: 1 in]
                  n303 = Exclusive Or(1:w1066, 2:w1064) -> (0:w1065:bool)
                  n304 = feedback-in #8(w1065) -> ()
                  n305 = global read "GlobalVI.vi" "emergencyStop"() -> (w1057:bool)
                  n306 = xnode "Running LED 5"("CommG"=w1064, "CommR"=TRUE) -> ("error out"=w1061:errorcluster)  [unwired: 1 in]
                  n307 = local read "liftState"() -> (w1059:i32)
                  n308 = Not Equal?(x=w1059, y=4 ("liftState")) -> (x != y?=w1058:bool)
                  n309 = Or(x=w1057, y=w1058) -> (x .or. y?=w1056:bool)
                  n310 = call "Time Delay12"("error in (no error)"=w1061, "Delay Time (s)"=0.25) -> ()  [unwired: 9 in, 1 out]
                }
                n311 = while {
                  stop <- w1045 stop-if-true
                  n312 = Tick Count (ms)() -> (millisecond timer value=w1051:u32)
                  n313 = local read "timerCount"() -> (w1050:u32)
                  n314 = Subtract(x=w1051, y=w1050) -> (x-y=w1042:u32)
                  n315 = Greater?(x=w1042, y=u32 10000) -> (0:w1043:bool)
                  n316 = local write "timeoutCounter"(w1042) -> ()
                  n317 = local write "timeoutError"(w1043) -> ()
                  n318 = global read "GlobalVI.vi" "emergencyStop"() -> (w1049:bool)
                  n319 = local read "liftState"() -> (w1047:i32)
                  n320 = Not Equal?(x=w1047, y=4 ("liftState")) -> (x != y?=w1048:bool)
                  n321 = Or(x=w1049, y=w1048) -> (x .or. y?=w1045:bool)
                }
                n322 = call "Motor_Controller.vi"("error in (no error)"=w1036, "stopMotors"=TRUE) -> ("error out"=w1035:errorcluster)  [unwired: 13 in]
                n323 = call "Time Delay 4"("error in (no error)"=w1035, "Delay Time (s)"=1.0) -> ("error out"=w1038:errorcluster)  [unwired: 9 in]
                n324 = case shown="False" w1039 {
                  tunnel: w1038 -> [_ _]
                  frame False {
                    n325 = local read "liftState"() -> (w1054:i32)
                    n326 = global write "GlobalVI.vi" "TrashCanOn"(TRUE ("TrashCanOn")) -> ()
                    n327 = Increment(x=w1054) -> (x+1=w1053:i32)
                    n328 = local write "liftState"(w1053) -> ()
                  }
                  frame True {
                    n329 = local write "liftState"(0 ("liftState")) -> ()
                  }
                }
              }
              frame 5 {
                # "The lift should not run anymore"
                # "Change back to default state"
                n330 = global write "GlobalVI.vi" "currentLiftState"(w1150) -> ()
                n331 = global write "GlobalVI.vi" "runLiftStatemachine"(FALSE ("runLiftStatemachine")) -> ()
                n332 = local write "liftState"(0 ("liftState")) -> ()
                n333 = Wait (ms)(milliseconds to wait=u32 1000) -> ()  [unwired: 1 out]
              }
            }
          }
        }
        n334 = global read "GlobalVI.vi" "emergencyStop"() -> (w54:bool)
        "timeoutError" <- FALSE ("timeoutError")
        "timeoutCounter" <- u32 0 ("timeoutCounter")
      }
    }
  }
  n335 = while {
    stop <- w1158 stop-if-true
    # "Status Updater"
    n336 = local read "timeoutError"() -> (w1161:bool)
    n337 = global read "GlobalVI.vi" "emergencyStop"() -> (w1158:bool)
    n338 = Not(x=w1161) -> (.not. x?=w1160:bool)
    n339 = global write "GlobalVI.vi" "liftStatus"(w1160) -> ()
    n340 = Wait Until Next ms Multiple(millisecond multiple=u32 200) -> ()  [unwired: 1 out]
    n341 = xnode "Digital input (1 sample) 2"() -> ("DIO/DIO2 (Pin 2)"=w1155:bool)  [unwired: 1 in, 1 out]
    n342 = xnode "Digital input (1 sample)"() -> ("DIO/DIO4 (Pin 4)"=w1153:bool)  [unwired: 1 in, 1 out]
    n343 = Not(x=w1155) -> (.not. x?=w1154:bool)
    "Trash can detection)" <- w1154
    n344 = Not(x=w1153) -> (.not. x?=w1152:bool)
    "DIO/DIO4 (Pin 4)" <- w1152
    n345 = global write "GlobalVI.vi" "runLiftStatemachine"("runLiftStatemachine") -> ()
    n346 = global write "GlobalVI.vi" "TrashCanDetection"(w1154) -> ()
    n347 = global read "GlobalVI.vi" "TrashCanOn"() -> (→"TrashCanOn":bool)
    n348 = global write "GlobalVI.vi" "emergencyStop"(w1152) -> ()
  }
